vi "Programa_robot_final_7.vi"(8 "error in (no error)":errorcluster) -> (0 "error out":errorcluster={"status"=FALSE, "code"=1073676294, "source"="VISA Read in Programa_robot_final_7.vi"} {"code" format="%f"})   [LabVIEW 2019]
uses:
  <vilib>/Instr/_visa.llb/VISA Configure Serial Port (Instr).vi
  Global_STOP.vi
  <vilib>/regexp/Match Regular Expression.xnode
panel:
  out "FIN BANDEJA ENTRADA":bool
  out "FIN BANDEJA OK":bool
  out "FIN BANDEJA NOK":bool
  out "NUMERO ASICS TESTEADOS":i32=8
  in  "stop socket 3":bool
  in  "Ruta hacia el fichero que contiene la imagen de la       superficie del ASIC  fotografiada por la camara en el bloque de borrado de la imagen previa capturada":path=path "C:/Trabajo_Robot/Test Asic Javi_2021/Origen Socket SERVO_PCB_BUENO_v5 (muchos asics)/capturaQR.jpg"
  in  "stop 6":bool
  in  "Abrir socket 2":bool
  in  "Cerrar socket 2":bool
  in  "Interruptor Error 2":bool
  in  "stop 5":bool
  out "Datos_QR 3":string
  out "Existe foto anterior?":bool
  in  "STOP TEST 3":bool
  in  "Interruptor Error":bool
  in  "Cerrar socket":bool
  in  "Abrir socket":bool
  out "Error_QR":bool=TRUE
  out "return count":u32=1
  out "lectura puerto serie":u32
  out "dato escrito puerto serie":string="0"
  out "TEST OK":bool
  in  "STOP TEST 2":bool
  out "Datos_QR 2":string
  in  "Config File":path=path "C:/Trabajo_Robot/Test Asic Javi_2021/Origen Socket SERVO_PCB_BUENO_v5 (muchos asics)/CONFIG/configuracion_robot_CTAV2022A.test"
  in  "SELECCION DE TEST":string(combo)="COMPLETO"
  in  "?":bool
  out "Boolean":bool
  in  "stop socket 2":bool
  out "Bytes at port 3":u32=1
  in  "IN y":string(combo)="00"
  in  "IN x":string(combo)="00"
  in  "NOK y":string(combo)="00"
  in  "NOK x":string(combo)="00"
  in  "OK y":string(combo)="00"
  in  "OK x":string(combo)="00"
  in  "Operator's name":string(combo)="Iñigo Jorge"
  in  "?":bool
  in  "Fichero de registro":path=path "C:/Trabajo_Robot/QC_LSTSUR/LOG/registro.txt"
  in  "Path Out Report":path=path "C:/Trabajo_Robot/QC_LSTSUR"
  in  "stop socket":bool
  out "Bytes at port 1":u32=1
  out "Iteraciones":i32=9
  out "Lectura buffer":string
  in  "Delay (ms)":dbl=1.0 min=1.0 max=9.0 step=1.0
  out "Bytes at port 2":u32
  in  "Interruptor":bool=TRUE
  in  "stop":bool
  # "SI EL TEST SE RALENTIZA, HAY QUE ABORTAR LABVIEW, PRESIONANDO\nEL BOTÓN DE ABORT, Y DESPUÉS SALIRSE COMPLETAMENTE DE LABVIEW, INCLUYENDO\nCERRAR LA VENTANA GENÉRICA DE LABVIEW QUE NOS SALE DESPUÉS DE QUE SE CIERRE\n\"PROGRAMA_ROBOT_FINAL_7\", PORQUE ES CUANDO LIBERA LA MEMORIA Y DESAPARECEN\nLAS SESIONES VISA y USB QUE NO SE HAN CERRADO AL ABORTAR.\n\nDESPUÉS HAY QUE REINICIAR ARDUINO, DESCONECTANDO Y CONECTANDO EL USB.\n\nCON ÉSTO YA SE PODRÍA VOLVER  A ABRIR EL \"PROGRAMA_ROBOT_FINAL_7\", CON TODO PARTIENDO DE CERO.\n\nEN CUALQUIER OTRA SITUACUÓN QUE PRESIONEMOS EL ABORT DE LABVIEW HAY QUE REALIZAR LA MISMA SECUENCIA."
  # "x: columna en cada bandeja \ny: fila en cada bandeja"
  # "Funcionamiento: en la primera iteración, el efector se desplaza desde el origen hasta la celda\nintroducida, hace una pausa, va a la posición del socket (0,0), hace otra pausa, va a la celda\nde salida y vuelve al origen. En las iteraciones siguientes hará lo mismo pero recorriendo las\nceldas de la bandeja sucesivamente. Que el desplazamiento se produzca hacia una celda de\nla bandeja OK o de la bandeja NOK depende de la salidad del programa de test de Asics."
types:
  T1 = enum16{"open", "replace", "create", "open or create", "replace or create", "replace or create with confirmation"}
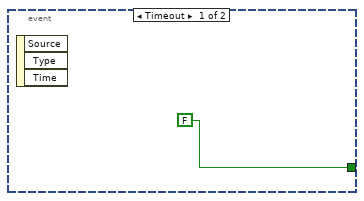
[diagram p2: hidden frame]
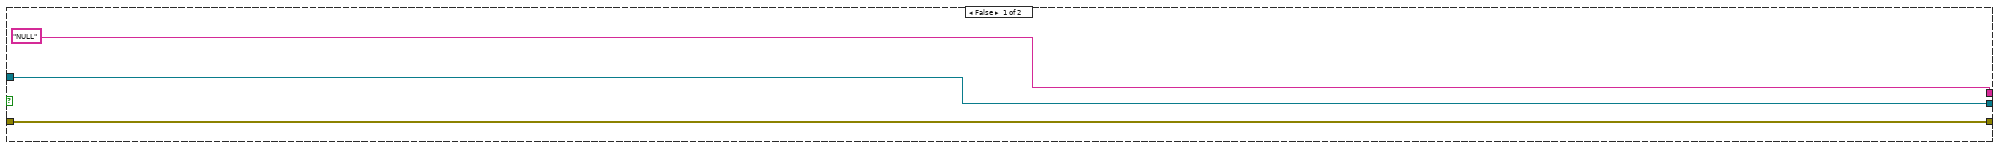
[diagram p5: hidden frame]
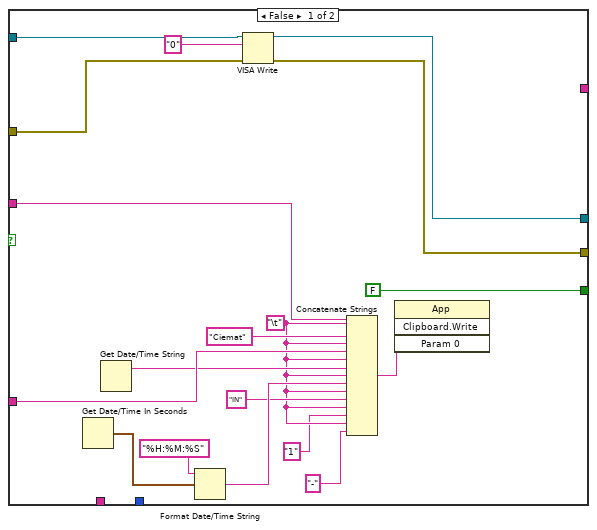
[diagram p9: hidden frame]
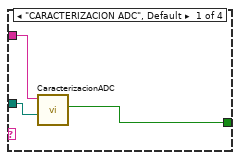
[diagram p10: hidden frame]
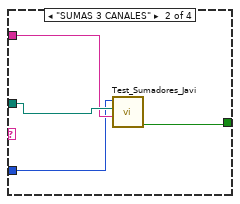
[diagram p11: hidden frame]
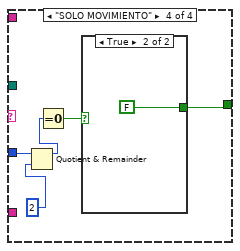
[diagram p12: hidden frame]
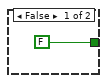
[diagram p13: hidden frame]
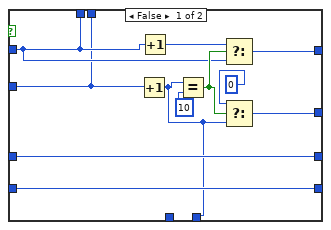
[diagram p15: hidden frame]
diagram:
  # "COORDENADA INICIAL DE \nLA BANDEJA DE ENTRADA"
  n1 = control-ref of="stop socket"() -> (w4:refnum<vi>)
  n2 = control-ref of="Cerrar socket"() -> (w12:refnum<vi>)
  n3 = control-ref of="STOP TEST 2"() -> (w15:refnum<vi>)
  n4 = control-ref of="Abrir socket"() -> (w10:refnum<vi>)
  n5 = control-ref of="stop"() -> (w11:refnum<vi>)
  n6 = control-ref of="Interruptor Error"() -> (w13:refnum<vi>)
  n7 = property class="Bool (strict)"(reference=w15, "Visible"=FALSE) -> ()  [unwired: 1 in, 2 out]
  n8 = property class="Bool (strict)"(reference=w10, "Visible"=FALSE) -> ()  [unwired: 1 in, 2 out]
  n9 = property class="Bool (strict)"(reference=w13, "Visible"=FALSE) -> ()  [unwired: 1 in, 2 out]
  n10 = property class="Bool (strict)"(reference=w12, "Visible"=FALSE) -> ()  [unwired: 1 in, 2 out]
  n11 = property on="Boolean" class="Bool (strict)"("Visible"=FALSE) -> ()  [unwired: 2 in, 2 out]
  n12 = property class="Bool"(reference=w4, "Visible"=FALSE) -> ()  [unwired: 1 in, 2 out]
  n13 = property class="Bool"(reference=w11, "Visible"=FALSE) -> ()  [unwired: 1 in, 2 out]
  n14 = flat-sequence {
    tunnel: [w60] -> w21
    tunnel: ["Fichero de registro"] -> w20
    tunnel: ["SELECCION DE TEST"] -> w19
    tunnel: ["NOK y"] -> w34
    tunnel: ["NOK x"] -> w33
    tunnel: ["OK y"] -> w32
    tunnel: ["OK x"] -> w31
    tunnel: ["IN y"] -> w30
    tunnel: ["IN x"] -> w29
    tunnel: [w63] -> w28
    tunnel: [w64] -> w27
    tunnel: ["IN y"] -> w26
    tunnel: ["IN x"] -> w25
    tunnel: w20 -> [w62]
    frame #0 {
      # "POLLING PARA DETECTAR LA PULSACION\nDEL BOTON DE START"
      n15 = while {
        stop <- "?" stop-if-true
        n16 = property class="Bool"("Visible"=TRUE) -> ()  [unwired: 2 in, 2 out]
        n17 = Not(x="?") -> (.not. x?=w55:bool)
        "Boolean" <- w55
        n18 = property on="Boolean" class="Bool (strict)"("Blinking"=w55) -> ()  [unwired: 2 in, 2 out]
      }
      n19 = property on="FIN BANDEJA ENTRADA" class="Bool (strict)"("Value"=FALSE ("FIN BANDEJA ENTRADA")) -> ()  [unwired: 2 in, 2 out]
      n20 = property on="FIN BANDEJA OK" class="Bool (strict)"("Value"=FALSE ("FIN BANDEJA OK")) -> ()  [unwired: 2 in, 2 out]
      n21 = property on="FIN BANDEJA NOK" class="Bool (strict)"("Value"=FALSE ("FIN BANDEJA NOK")) -> ()  [unwired: 2 in, 2 out]
      n22 = global write "Global_STOP.vi" "stop"(FALSE ("stop")) -> ()
    }
    frame #1 {
      # "BOTON START DESAPARECE"
      n23 = property class="Bool"("Visible"=FALSE) -> ()  [unwired: 2 in, 2 out]
      n24 = Not(x="?") -> (.not. x?=w60:bool)
    }
    frame #2 {
      # "abre el fichero de log donde se registra los asics testeados , resultado del test\noperador , fila y columna de la bandeja donde ha cogido asic , fecha..."
      n25 = Open/Create/Replace File(file path (use dialog)=w62, operation (0:open)=T1."open or create", access (0:read/write)=enum16{"read/write", "read-only", "write-only"}."write-only") -> (refnum out=w75:refnum<file>, error out=w77:errorcluster)  [unwired: 3 in, 1 out]
      n26 = Set File Position(refnum=w75, from (0:start)=enum16{"start", "end", "current"}."end", error in=w77) -> (refnum out=w76:refnum<file>, error out=w78:errorcluster)  [unwired: 1 in]
      n27 = Write to Text File(file (use dialog)=w76, text="\r\n", error in=w78) -> (refnum out=w64:refnum<file>, error out=w63:errorcluster)  [unwired: 1 in, 1 out]
    }
  }
  n28 = Decimal String To Number(string=w26) -> (number=w3:i32)  [unwired: 2 in, 1 out]
  n29 = Decimal String To Number(string=w25) -> (number=w2:i32)  [unwired: 2 in, 1 out]
  n30 = Multiply(x=10, y=w3) -> (x*y=w23:i32)
  n31 = Decimal String To Number(string=w32) -> (number=w36:i32)  [unwired: 2 in, 1 out]
  n32 = Decimal String To Number(string=w31) -> (number=w35:i32)  [unwired: 2 in, 1 out]
  n33 = Decimal String To Number(string=w34) -> (number=w38:i32)  [unwired: 2 in, 1 out]
  n34 = Decimal String To Number(string=w33) -> (number=w37:i32)  [unwired: 2 in, 1 out]
  n35 = call-poly "VISA Configure Serial Port"("VISA resource name"=refnum<visa-resource-name> "COM4", "baud rate (9600)"=u32 9600, "data bits (8)"=u16 8, "error in (no error)"="error in (no error)") -> ("VISA resource name out"=w42:refnum<visa-resource-name>, "error out"=w45:errorcluster)  [unwired: 10 in]
  n36 = Add(x=w23, y=w2) -> (x+y=w22:i32)
  n37 = while {
    shift-right: [w121] -> w43
    shift-left: w45 -> [w156]
    tunnel: w42 -> [w154]
    tunnel: [w123] -> w44
    tunnel: w27 -> [w147]
    tunnel: [w146] -> w41
    tunnel: w28 -> [w145]
    tunnel: [w144] -> w40
    tunnel: w29 -> [w142]
    tunnel: w30 -> [w141]
    tunnel: w31 -> [w140]
    tunnel: w32 -> [w139]
    tunnel: w33 -> [w138]
    tunnel: w34 -> [w137]
    shift-right: [w105] -> _
    shift-left: w38 -> [w136]
    shift-right: [w102] -> _
    shift-left: w37 -> [w135]
    shift-right: [w104] -> _
    shift-left: w36 -> [w134]
    shift-right: [w101] -> _
    shift-left: w35 -> [w133]
    tunnel: w22 -> [w111]
    tunnel: w21 -> [w125]
    tunnel: w19 -> [w124]
    tunnel: [w112] -> w17
    shift-right: [w79] -> _
    shift-left: w3 -> [w89]
    shift-right: [w80] -> _
    shift-left: w2 -> [w88]
    i -> [w109]
    stop <- w110 stop-if-true
    w100 = 10
    w103 = 26 ("y")
    # "Cuando Arduino deja un ASIC en la bandeja de  entrada ó en las de OK/NOK\ny vuelve a la posicion de socket, envia un \"2\" por el puerto serie\na labview y éste lo lee para que se salga del bucle, y prosiga la secuencia que le queda\nal programa, para después coger otro asic. Javier Morales"
    n38 = flat-sequence {
      tunnel: w156 -> [w211]
      tunnel: w154 -> [w200]
      tunnel: [w202] -> w153
      tunnel: [w201] -> w152
      tunnel: w142 -> [w181]
      tunnel: w141 -> [w180]
      tunnel: w140 -> [w179]
      tunnel: w139 -> [w178]
      tunnel: w138 -> [w177]
      tunnel: w137 -> [w176]
      tunnel: w153 -> [w948]
      tunnel: w152 -> [w947]
      tunnel: [w946] -> w132
      tunnel: [w945] -> w130
      tunnel: [w944] -> _
      tunnel: w132 -> [w965]
      tunnel: [w963] -> w131
      tunnel: w130 -> [w964]
      tunnel: [w962] -> w129
      tunnel: w131 -> [w987]
      tunnel: w129 -> [w986]
      tunnel: w109 -> [w988]
      tunnel: [w984] -> w128
      tunnel: [w983] -> w127
      tunnel: [w982] -> w126
      tunnel: [w979] -> w107
      tunnel: w109 -> [w1106]
      tunnel: [w1108] -> w150
      tunnel: [w1107] -> w149
      tunnel: [w1104] -> w143
      tunnel: w128 -> [w1103]
      tunnel: w127 -> [w1102]
      tunnel: w126 -> [w1101]
      tunnel: w125 -> [w1096]
      tunnel: w124 -> [w1099]
      tunnel: w109 -> [w1098]
      tunnel: [w1092] -> w108
      tunnel: w107 -> [w1092]
      tunnel: [w1091] -> w106
      tunnel: [w1190] -> w148
      tunnel: [w1192] -> w151
      tunnel: w150 -> [w1191]
      tunnel: w149 -> [w1189]
      tunnel: w147 -> [w1196]
      tunnel: [w1195] -> w146
      tunnel: w145 -> [w1194]
      tunnel: [w1193] -> w144
      tunnel: w109 -> [w1186]
      tunnel: w143 -> [w1185]
      tunnel: w136 -> [w1181]
      tunnel: w135 -> [w1184]
      tunnel: w134 -> [w1183]
      tunnel: w133 -> [w1182]
      tunnel: [w1180] -> w105
      tunnel: [w1179] -> w102
      tunnel: [w1178] -> w104
      tunnel: [w1177] -> w101
      tunnel: w111 -> [w1176]
      tunnel: w109 -> [w1175]
      tunnel: [w1174] -> _
      tunnel: w108 -> [w1173]
      tunnel: w106 -> [w1172]
      tunnel: [w1171] -> w93
      tunnel: [w1170] -> w92
      tunnel: w89 -> [w1164]
      tunnel: w88 -> [w1169]
      tunnel: [w1166] -> w80
      tunnel: [w1162] -> w79
      tunnel: [w1161] -> w86
      frame #0 {
        n39 = for {
          N: 2 -> [_]
          shift-right: [w823] -> _
          shift-left: w181 -> [w828]
          shift-right: [w826] -> w197
          shift-left: w200 -> [w827]
          shift-right: [w824] -> w196
          shift-left: w211 -> [w825]
          n40 = xnode "Match Regular Expression"("input string"=w828, "regular expression"="-?\\d") -> ("whole match"=w822:string, "after match"=w823:string)  [unwired: 4 in, 3 out]
          n41 = VISA Write(VISA resource name=w827, write buffer=w822, error in (no error)=w825) -> (VISA resource name out=w826:refnum<visa-resource-name>, error out=w824:errorcluster)  [unwired: 1 out]
        }
        n42 = for {
          N: 2 -> [_]
          shift-right: [w701] -> _
          shift-left: w180 -> [w706]
          shift-right: [w704] -> w191
          shift-left: w197 -> [w705]
          shift-right: [w702] -> w190
          shift-left: w196 -> [w703]
          n43 = xnode "Match Regular Expression"("input string"=w706, "regular expression"="-?\\d") -> ("whole match"=w700:string, "after match"=w701:string)  [unwired: 4 in, 3 out]
          n44 = VISA Write(VISA resource name=w705, write buffer=w700, error in (no error)=w703) -> (VISA resource name out=w704:refnum<visa-resource-name>, error out=w702:errorcluster)  [unwired: 1 out]
        }
        n45 = for {
          N: 2 -> [_]
          shift-right: [w579] -> _
          shift-left: w179 -> [w584]
          shift-right: [w582] -> w193
          shift-left: w191 -> [w583]
          shift-right: [w580] -> w192
          shift-left: w190 -> [w581]
          n46 = xnode "Match Regular Expression"("input string"=w584, "regular expression"="-?\\d") -> ("whole match"=w578:string, "after match"=w579:string)  [unwired: 4 in, 3 out]
          n47 = VISA Write(VISA resource name=w583, write buffer=w578, error in (no error)=w581) -> (VISA resource name out=w582:refnum<visa-resource-name>, error out=w580:errorcluster)  [unwired: 1 out]
        }
        n48 = for {
          N: 2 -> [_]
          shift-right: [w457] -> _
          shift-left: w178 -> [w462]
          shift-right: [w460] -> w185
          shift-left: w193 -> [w461]
          shift-right: [w458] -> w184
          shift-left: w192 -> [w459]
          n49 = xnode "Match Regular Expression"("input string"=w462, "regular expression"="-?\\d") -> ("whole match"=w456:string, "after match"=w457:string)  [unwired: 4 in, 3 out]
          n50 = VISA Write(VISA resource name=w461, write buffer=w456, error in (no error)=w459) -> (VISA resource name out=w460:refnum<visa-resource-name>, error out=w458:errorcluster)  [unwired: 1 out]
        }
        n51 = for {
          N: 2 -> [_]
          shift-right: [w335] -> _
          shift-left: w177 -> [w340]
          shift-right: [w338] -> w187
          shift-left: w185 -> [w339]
          shift-right: [w336] -> w186
          shift-left: w184 -> [w337]
          n52 = xnode "Match Regular Expression"("input string"=w340, "regular expression"="-?\\d") -> ("whole match"=w334:string, "after match"=w335:string)  [unwired: 4 in, 3 out]
          n53 = VISA Write(VISA resource name=w339, write buffer=w334, error in (no error)=w337) -> (VISA resource name out=w338:refnum<visa-resource-name>, error out=w336:errorcluster)  [unwired: 1 out]
        }
        n54 = for {
          N: 2 -> [_]
          shift-right: [w213] -> _
          shift-left: w176 -> [w218]
          shift-right: [w216] -> w183
          shift-left: w187 -> [w217]
          shift-right: [w214] -> w182
          shift-left: w186 -> [w215]
          n55 = xnode "Match Regular Expression"("input string"=w218, "regular expression"="-?\\d") -> ("whole match"=w212:string, "after match"=w213:string)  [unwired: 4 in, 3 out]
          n56 = VISA Write(VISA resource name=w217, write buffer=w212, error in (no error)=w215) -> (VISA resource name out=w216:refnum<visa-resource-name>, error out=w214:errorcluster)  [unwired: 1 out]
        }
        n57 = Number To Decimal String(number="Delay (ms)") -> (decimal integer string=w205:string)  [unwired: 1 in]
        n58 = VISA Write(VISA resource name=w183, write buffer=w205, error in (no error)=w182) -> (VISA resource name out=w207:refnum<visa-resource-name>, error out=w206:errorcluster)  [unwired: 1 out]
        n59 = Select(t="1" ("write buffer"), s="Interruptor", f="0" ("write buffer")) -> (s? t:f=w203:string)
        n60 = VISA Write(VISA resource name=w207, write buffer=w203, error in (no error)=w206) -> (VISA resource name out=w202:refnum<visa-resource-name>, error out=w201:errorcluster)  [unwired: 1 out]
      }
      frame #1 {
        n61 = while {
          shift-right: [w955] -> w945
          shift-left: w947 -> [w960]
          tunnel: ["stop socket"] -> _
          shift-right: [w956] -> w946
          shift-left: w948 -> [w961]
          tunnel: ["stop socket"] -> w944
          stop <- w950 stop-if-true
          n62 = property class="Instr"(reference=w961, error in=w960) -> (reference out=w959:refnum<visa-resource-name>, error out=w958:errorcluster, "Bytes at Port"=w957:u32)
          "Bytes at port 1" <- w957
          n63 = VISA Read(VISA resource name=w959, byte count=w957, error in (no error)=w958) -> (VISA resource name out=w956:refnum<visa-resource-name>, read buffer=w954:string, error out=w955:errorcluster)  [unwired: 1 out]
          n64 = Equal?(x="2", y=w954) -> (x = y?=w952:bool)
          n65 = global read "Global_STOP.vi" "stop"() -> (w949:bool)
          n66 = Compound Arithmetic op=OR(w952, "stop socket", w949) -> (w950:bool)
        }
      }
      frame #2 {
        n67 = while {
          shift-right: [w972] -> w962
          shift-left: w964 -> [w977]
          tunnel: ["stop socket 2"] -> _
          shift-right: [w973] -> w963
          shift-left: w965 -> [w978]
          tunnel: ["stop socket 2"] -> _
          stop <- w967 stop-if-true
          n68 = property class="Instr"(reference=w978, error in=w977) -> (reference out=w976:refnum<visa-resource-name>, error out=w975:errorcluster, "Bytes at Port"=w974:u32)
          "Bytes at port 3" <- w974
          n69 = VISA Read(VISA resource name=w976, byte count=w974, error in (no error)=w975) -> (VISA resource name out=w973:refnum<visa-resource-name>, read buffer=w971:string, error out=w972:errorcluster)  [unwired: 1 out]
          n70 = Equal?(x="3", y=w971) -> (x = y?=w969:bool)
          n71 = global read "Global_STOP.vi" "stop"() -> (w966:bool)
          n72 = Compound Arithmetic op=OR(w969, "stop socket 2", w966) -> (w967:bool)
        }
      }
      frame #3 {
        # "Este bloque realiza la captura y lectura del QR"
        n73 = Greater?(x=w988, y=-1) -> (0:w985:bool)
        n74 = case shown="True" w985 {
          tunnel: [w992 w995] -> w982
          tunnel: w987 -> [w992 w997]
          tunnel: [w991 w996] -> w984
          tunnel: w986 -> [w991 w998]
          tunnel: ["NULL" ("Datos_QR") w994] -> w983
          frame False {
          }
          frame True {
            n75 = property on="Error_QR" class="Bool (strict)"("Value"=FALSE ("Error_QR")) -> ()  [unwired: 2 in, 2 out]
            n76 = while {
              tunnel: [w1005] -> w994
              tunnel: w997 -> [w1015]
              tunnel: [w1011] -> w995
              tunnel: [w1010] -> w996
              tunnel: w998 -> [w1006]
              stop <- w1003 stop-if-true
              n77 = flat-sequence {
                tunnel: [w1019] -> w1007
                tunnel: w1006 -> [w1017]
                tunnel: [w1031] -> w1005
                tunnel: [w1030] -> w1000
                tunnel: w1007 -> [w1029]
                tunnel: [w1029] -> w1001
                frame #0 {
                  # "Éste bloque borra el fichero de imagen\ndel Asic anterior."
                  n78 = call <vilib>:"Check if File or Folder Exists.vi"("error in (no error)"=w1017, "path"="Ruta hacia el fichero que contiene la imagen de la       superficie del ASIC  fotografiada por la camara en el bloque de borrado de la imagen previa capturada") -> ("error out"=w1018:errorcluster, "file or folder exists?"=w1021:bool, "dup path"=w1020:path)  [unwired: 7 in]
                  "Existe foto anterior?" <- w1021
                  n79 = case shown="True" w1021 {
                    tunnel: w1020 -> [w1023 w1027]
                    tunnel: [w1023 w1026] -> _
                    tunnel: [w1022 w1025] -> w1019
                    tunnel: w1018 -> [w1022 w1024]
                    frame False {
                    }
                    frame True {
                      n80 = Delete(path (use dialog)=w1027, error in=w1024) -> (deleted path=w1026:path, error out=w1025:errorcluster)  [unwired: 3 in, 1 out]
                    }
                  }
                }
                frame #1 {
                  # "Éste bloque realiza la captura de imagen\ndel QR del Asic para leer el código."
                  n81 = for {
                    N: 5 -> [_]
                    tunnel: [w1036] -> w1031
                    tunnel: [w1034] -> w1030
                    stop <- w1032 stop-if-true
                    n82 = call "CapturaImagenyQR_subVI_pruebas.vi"() -> ("Datos_QR"=w1036:string)  [unwired: 11 in]
                    "Datos_QR 3" <- w1036
                    n83 = Equal?(x=w1036, y="" ("Datos_QR")) -> (x = y?=w1035:bool)
                    n84 = global read "Global_STOP.vi" "stop"() -> (w1033:bool)
                    n85 = Not(x=w1035) -> (.not. x?=w1034:bool)
                    n86 = Compound Arithmetic op=OR(w1034, w1033) -> (w1032:bool)
                  }
                }
              }
              n87 = Not(x=w1000) -> (.not. x?=w1002:bool)
              "Error_QR" <- w1002
              n88 = Select(t="1" ("write buffer"), s=w1000, f="0" ("write buffer")) -> (s? t:f=w1012:string)
              n89 = VISA Write(VISA resource name=w1015, write buffer=w1012, error in (no error)=w1001) -> (VISA resource name out=w1009:refnum<visa-resource-name>, error out=w1008:errorcluster)  [unwired: 1 out]
              n90 = global read "Global_STOP.vi" "stop"() -> (w1004:bool)
              n91 = case shown="False" w1000 {
                tunnel: w1009 -> [w1049 w1090]
                tunnel: w1008 -> [w1048 w1089]
                tunnel: [w1047 w1090] -> w1011
                tunnel: [w1046 w1089] -> w1010
                frame False {
                  n92 = flat-sequence {
                    tunnel: w1049 -> [w1053]
                    tunnel: [w1052] -> w1045
                    tunnel: [w1051] -> w1043
                    tunnel: w1048 -> [w1050]
                    tunnel: w1045 -> [w1066]
                    tunnel: [w1066] -> w1044
                    tunnel: w1043 -> [w1065]
                    tunnel: [w1065] -> w1042
                    tunnel: w1044 -> [w1070]
                    tunnel: w1042 -> [w1069]
                    tunnel: [w1068] -> w1041
                    tunnel: [w1067] -> w1039
                    tunnel: w1041 -> [w1083]
                    tunnel: [w1083] -> w1040
                    tunnel: w1039 -> [w1082]
                    tunnel: [w1082] -> w1038
                    tunnel: [w1084] -> w1046
                    tunnel: [w1085] -> w1047
                    tunnel: w1040 -> [w1085]
                    tunnel: w1038 -> [w1084]
                    frame #0 {
                      n93 = while {
                        tunnel: w1053 -> [w1063]
                        tunnel: [w1059] -> w1052
                        tunnel: [w1058] -> w1051
                        tunnel: w1050 -> [w1057]
                        stop <- w1054 stop-if-true
                        n94 = global read "Global_STOP.vi" "stop"() -> (w1056:bool)
                        n95 = Select(t="2" ("write buffer"), s="Abrir socket", f="0" ("write buffer")) -> (s? t:f=w1060:string)
                        n96 = Or(x=w1056, y="Abrir socket") -> (x .or. y?=w1054:bool)
                        n97 = VISA Write(VISA resource name=w1063, write buffer=w1060, error in (no error)=w1057) -> (VISA resource name out=w1059:refnum<visa-resource-name>, error out=w1058:errorcluster)  [unwired: 1 out]
                      }
                    }
                    frame #1 {
                      n98 = Wait (ms)(milliseconds to wait=u32 1000) -> ()  [unwired: 1 out]
                    }
                    frame #2 {
                      n99 = while {
                        tunnel: w1070 -> [w1077]
                        tunnel: w1069 -> [w1076]
                        tunnel: [w1075] -> w1068
                        tunnel: [w1074] -> w1067
                        stop <- w1073 stop-if-true
                        n100 = global read "Global_STOP.vi" "stop"() -> (w1072:bool)
                        n101 = Select(t="3" ("write buffer"), s="Cerrar socket", f="0" ("write buffer")) -> (s? t:f=w1078:string)
                        n102 = Or(x=w1072, y="Cerrar socket") -> (x .or. y?=w1073:bool)
                        n103 = VISA Write(VISA resource name=w1077, write buffer=w1078, error in (no error)=w1076) -> (VISA resource name out=w1075:refnum<visa-resource-name>, error out=w1074:errorcluster)  [unwired: 1 out]
                      }
                    }
                    frame #3 {
                      n104 = Wait (ms)(milliseconds to wait=u32 1000) -> ()  [unwired: 1 out]
                    }
                    frame #4 {
                      n105 = while {
                        stop <- w1086 stop-if-true
                        n106 = global read "Global_STOP.vi" "stop"() -> (w1088:bool)
                        n107 = Or(x="Interruptor Error", y=w1088) -> (x .or. y?=w1086:bool)
                      }
                    }
                  }
                }
                frame True {
                }
              }
              n108 = Or(x=w1000, y=w1004) -> (x .or. y?=w1003:bool)
              n109 = case shown="True" w1002 {
                frame False {
                }
                frame True {
                  n110 = call "Send Email"() -> ()  [unwired: 11 in, 1 out]
                }
              }
            }
            n111 = Wait (ms)(milliseconds to wait=u32 10000) -> ()  [unwired: 1 out]
          }
        }
        n112 = control-ref of="STOP TEST 2"() -> (w981:refnum<vi>)
        n113 = property class="Bool (strict)"(reference=w981, "Visible"=TRUE) -> ()  [unwired: 1 in, 2 out]
        n114 = Get Date/Time In Seconds() -> (seconds since 1Jan1904=w979:timestamp)
      }
      frame #4 {
        n115 = global read "Global_STOP.vi" "stop"() -> (w1095:bool)
        n116 = Greater?(x=w1106, y=-1) -> (0:w1097:bool)
        n117 = Not(x=w1095) -> (.not. x?=w1094:bool)
        n118 = Compound Arithmetic op=AND(w1097, w1096, w1094) -> (w1093:bool)
        n119 = case shown="True" w1093 {
          tunnel: w1101 -> [w1124 w1133]
          tunnel: w1103 -> [w1123 w1132]
          tunnel: [w1122 w1131] -> w1108
          tunnel: [w1121 w1130] -> w1107
          tunnel: w1102 -> [w1117 w1127]
          tunnel: [FALSE ("Boolean") w1137] -> w1104
          tunnel: "Operator's name" -> [w1115 w1136]
          tunnel: w1099 -> [_ w1128]
          tunnel: w1098 -> [_ w1135]
          tunnel: [_ w1127] -> w1091
          frame False {
            w1111 = "\t"
            n120 = Get Date/Time In Seconds() -> (seconds since 1Jan1904=w1119:timestamp)
            n121 = Get Date/Time String() -> (date string=w1114:string)  [unwired: 3 in, 1 out]
            n122 = Format Date/Time String(time format string (%c)="%H:%M:%S", seconds (now)=w1119) -> (date/time string=w1113:string)  [unwired: 1 in]
            n123 = VISA Write(VISA resource name=w1124, write buffer="0", error in (no error)=w1123) -> (VISA resource name out=w1122:refnum<visa-resource-name>, error out=w1121:errorcluster)  [unwired: 1 out]
            n124 = Concatenate Strings(w1117, w1111, "Ciemat", w1111, w1115, w1111, w1114, w1111, w1113, w1111, "IN", w1111, "1", w1111, "-") -> (w1120:string)
            n125 = invoke class="App" method="Clipboard.Write"("Param 0"=w1120) -> ()  [unwired: 3 in, 4 out]
          }
          frame True {
            # "Test de Asics"
            n126 = case shown="\"COMPLETO\"" w1128 {
              tunnel: w1127 -> [w1143 w1145 w1153 _]
              tunnel: "Path Out Report" -> [w1142 w1147 w1151 _]
              tunnel: [w1141 w1146 w1149 w1154] -> w1137
              tunnel: w1136 -> [_ _ w1152 _]
              tunnel: w1135 -> [_ w1144 w1148 w1158]
              frame "CARACTERIZACION ADC", Default {
                n127 = call "CaracterizacionADC.vi"("QR code"=w1143, "Path Out Report"=w1142) -> ("OK/NOK"=w1141:bool)  [unwired: 7 in]
              }
              frame "SUMAS 3 CANALES" {
                n128 = call "Test_Sumadores_Javi.vi"("QR"=w1145, "Path"=w1147, "NUMERO DE PASADA DE TEST"=w1144) -> ("Boolean"=w1146:bool)  [unwired: 8 in]
              }
              frame "COMPLETO" {
                n129 = call "Test Asic V1.0_2019_2.vi"("Config File"="Config File", "Path Out Report"=w1151, "Operator's Name"=w1152, "ASIC'S Number"=w1153) -> ("OK, Fault 2"=w1149:bool)  [unwired: 1 in]
                "NUMERO ASICS TESTEADOS" <- w1148
              }
              frame "SOLO MOVIMIENTO" {
                n130 = Quotient & Remainder(x=w1158, y=2) -> (x-y*floor(x/y)=w1155:i32)  [unwired: 1 out]
                n131 = Equal To 0?(x=w1155) -> (x = 0?=w1156:bool)
                n132 = case shown="True" w1156 {
                  tunnel: [FALSE FALSE] -> w1154
                  frame False {
                  }
                  frame True {
                  }
                }
              }
            }
            "TEST OK" <- w1137
            n133 = Select(t="1" ("write buffer"), s=w1137, f="0" ("write buffer")) -> (s? t:f=w1134:string)
            "dato escrito puerto serie" <- w1134
            n134 = VISA Write(VISA resource name=w1133, write buffer=w1134, error in (no error)=w1132) -> (VISA resource name out=w1131:refnum<visa-resource-name>, return count=→"return count":u32, error out=w1130:errorcluster)
          }
        }
      }
      frame #5 {
        n135 = Greater?(x=w1186, y=-1) -> (0:w1187:bool)
        n136 = case shown="True" w1187 {
          tunnel: w1196 -> [w1202 w1207]
          tunnel: [w1202 w1208] -> w1195
          tunnel: w1194 -> [w1201 w1210]
          tunnel: [w1201 w1209] -> w1193
          tunnel: [w1204 w1228] -> w1192
          tunnel: w1191 -> [w1204 w1228]
          tunnel: [w1203 w1227] -> w1190
          tunnel: w1189 -> [w1203 w1227]
          tunnel: w1185 -> [_ w1213]
          tunnel: w1181 -> [w1200 w1226]
          tunnel: w1184 -> [w1199 w1225]
          tunnel: w1183 -> [w1198 w1224]
          tunnel: w1182 -> [w1197 w1223]
          tunnel: [w1200 w1222] -> w1180
          tunnel: [w1199 w1221] -> w1179
          tunnel: [w1198 w1220] -> w1178
          tunnel: [w1197 w1219] -> w1177
          tunnel: [_ w1214] -> _
          tunnel: w1173 -> [_ w1214]
          tunnel: w1172 -> [_ w1211]
          tunnel: [_ w1206] -> w1171
          tunnel: [_ w1205] -> w1170
          frame False {
          }
          frame True {
            # "Registro de datos en fichero"
            n137 = property on="Operator's name" class="CmbBox"() -> ("Value"=w1212:string)  [unwired: 2 in, 2 out]
            n138 = case shown="True" w1213 {
              tunnel: w1226 -> [w1231 w1244]
              tunnel: w1225 -> [w1230 w1243]
              tunnel: w1224 -> [w1233 w1241]
              tunnel: w1223 -> [w1232 w1242]
              tunnel: [w1235 w1244] -> w1222
              tunnel: [w1234 w1243] -> w1221
              tunnel: [w1233 w1246] -> w1220
              tunnel: [w1232 w1245] -> w1219
              tunnel: [w1231 w1241] -> w1218
              tunnel: [w1230 w1242] -> w1217
              tunnel: [_ w1240] -> w1206
              tunnel: [w1229 _] -> w1205
              frame False {
                n139 = Increment(x=w1230) -> (x+1=w1229:i32)
                n140 = Increment(x=w1231) -> (x+1=w1236:i32)
                n141 = Equal?(x=w1229, y=10) -> (x = y?=w1237:bool)
                n142 = Select(t=w1236, s=w1237, f=w1231) -> (s? t:f=w1235:i32)
                n143 = Select(t=0, s=w1237, f=w1229) -> (s? t:f=w1234:i32)
              }
              frame True {
                n144 = Increment(x=w1242) -> (x+1=w1240:i32)
                n145 = Increment(x=w1241) -> (x+1=w1247:i32)
                n146 = Equal?(x=w1240, y=10) -> (x = y?=w1248:bool)
                n147 = Select(t=w1247, s=w1248, f=w1241) -> (s? t:f=w1246:i32)
                n148 = Select(t=0, s=w1248, f=w1240) -> (s? t:f=w1245:i32)
              }
            }
            n149 = Number To Decimal String(number=w1218) -> (decimal integer string=w1216:string)  [unwired: 1 in]
            n150 = Number To Decimal String(number=w1217) -> (decimal integer string=w1215:string)  [unwired: 1 in]
            n151 = call "Escribir_Fichero_Registro.vi"("refnum FILE"=w1207, "ASIC QR CODE"=w1211, "HORA COMIENZO"=w1214, "Coordenada X"=w1215, "Coordenada Y"=w1216, "OPERADOR"=w1212, "Resultado test"=w1213, "error in (no error)"=w1210) -> ("refnum out"=w1208:refnum<file>, "error out"=w1209:errorcluster)  [unwired: 18 in]
          }
        }
        n152 = Increment(x=w1164) -> (x+1=w1165:i32)
        n153 = Increment(x=w1169) -> (x+1=w1161:i32)
        n154 = Equal?(x=w1161, y=10) -> (x = y?=w1163:bool)
        n155 = Select(t=i16 0, s=w1163, f=w1161) -> (s? t:f=w1166:i32)
        n156 = Select(t=w1165, s=w1163, f=w1164) -> (s? t:f=w1162:i32)
        n157 = Add(x=w1176, y=w1175) -> (x+y=w1174:i32)
      }
    }
    n158 = while {
      shift-right: [w1258] -> w116
      shift-left: w148 -> [w1264]
      tunnel: ["stop"] -> _
      shift-right: [w1259] -> w123
      shift-left: w151 -> [w1265]
      tunnel: [w1254] -> w155
      stop <- w1252 stop-if-true
      # "1"
      n159 = property class="Instr"(reference=w1265, error in=w1264) -> (reference out=w1262:refnum<visa-resource-name>, error out=w1261:errorcluster, "Bytes at Port"=w1260:u32)
      "Bytes at port 2" <- w1260
      n160 = VISA Read(VISA resource name=w1262, byte count=w1260, error in (no error)=w1261) -> (VISA resource name out=w1259:refnum<visa-resource-name>, read buffer=w1254:string, return count=w1257:u32, error out=w1258:errorcluster)
      "lectura puerto serie" <- w1257
      n161 = Greater Or Equal?(x=w1257, y=u32 1) -> (x >= y?=w1255:bool)
      n162 = global read "Global_STOP.vi" "stop"() -> (w1251:bool)
      n163 = Or(x=w1255, y="stop") -> (x .or. y?=w1253:bool)
      n164 = Compound Arithmetic op=OR(w1253, w1251) -> (w1252:bool)
    }
    "Lectura buffer" <- w155
    n165 = Equal?(x=w104, y=w103) -> (x = y?=w97:bool)
    n166 = Equal?(x=w105, y=w103) -> (x = y?=w99:bool)
    n167 = Equal?(x=w92, y=w100) -> (x = y?=w98:bool)
    n168 = Equal?(x=w93, y=w100) -> (x = y?=w96:bool)
    n169 = Equal?(x=w79, y=26) -> (x = y?=w84:bool)
    n170 = Equal?(x=w86, y=10) -> (x = y?=w83:bool)
    n171 = And(x=w99, y=w98) -> (x .and. y?=w95:bool)
    "FIN BANDEJA NOK" <- w95
    n172 = And(x=w84, y=w83) -> (x .and. y?=w82:bool)
    "FIN BANDEJA ENTRADA" <- w82
    n173 = And(x=w97, y=w96) -> (x .and. y?=w94:bool)
    "FIN BANDEJA OK" <- w94
    n174 = Or(x=w95, y=w94) -> (x .or. y?=w90:bool)
    n175 = flat-sequence {
      tunnel: w116 -> [w158]
      tunnel: [w158] -> w115
      tunnel: [w157] -> w113
      frame #0 {
        n176 = global read "Global_STOP.vi" "stop"() -> (w157:bool)
      }
    }
    n177 = case shown="False" w113 {
      selector: w113 -> [_ w168]
      tunnel: [w162 _] -> w120
      tunnel: [w159 w168] -> w117
      tunnel: w115 -> [w160 w167]
      tunnel: [w160 w167] -> w114
      frame False {
        n178 = for {
          N: 3 -> [_]
          tunnel: [w165] -> _
          tunnel: [w163] -> w162
          tunnel: [w163] -> w159
          stop <- w163 stop-if-true
          n179 = call "CapturaImagenyQR_subVI_pruebas.vi"() -> ("Datos_QR"=w165:string)  [unwired: 11 in]
          "Datos_QR 2" <- w165
          n180 = Equal?(x=w165, y="" ("Datos_QR")) -> (x = y?=w164:bool)
          n181 = Not(x=w164) -> (.not. x?=w163:bool)
        }
      }
      frame True {
      }
    }
    n182 = flat-sequence {
      tunnel: [w173] -> w112
      tunnel: w117 -> [w171]
      tunnel: [w170] -> w91
      tunnel: w90 -> [w170]
      tunnel: w82 -> [w169]
      tunnel: [w169] -> w81
      frame #0 {
        n183 = global read "Global_STOP.vi" "stop"() -> (w172:bool)
        n184 = Or(x=w171, y=w172) -> (x .or. y?=w173:bool)
      }
    }
    n185 = Boolean To (0,1)(Boolean=w120) -> (0, 1=w119:i16)
    n186 = call <vilib>:"Error Cluster From Error Code.vi"("error in (no error)"=w114, "error message (\"\")"="El asic no se ha colocado en la\n    bandeja de salida,se ha quedado\nen el socket posiblemente por una\nmala succión de la ventosa.\nPresione STOP\n" ("error message (\"\")"), "error code (0)"=w119) -> ("error out"=w118:errorcluster)  [unwired: 6 in]
    n187 = call <vilib>:"Simple Error Handler.vi"("error in (no error)"=w118) -> ("error out"=w121:errorcluster)  [unwired: 4 in, 4 out]
    n188 = Compound Arithmetic op=OR(w112, w91, w81) -> (w110:bool)
    n189 = case shown="True" w120 {
      selector: w120 -> [w174 w175]
      tunnel: [w174 w175] -> _
      frame False {
      }
      frame True {
        n190 = call "Send Email2"() -> ()  [unwired: 11 in, 1 out]
      }
    }
    "Iteraciones" <- w109
  }
  n191 = flat-sequence {
    frame #0 {
      n192 = local write "STOP TEST 2"(FALSE ("STOP TEST 2")) -> ()
    }
    frame #1 {
      n193 = while {
        stop <- w1267 stop-if-true
        n194 = event shown="[1] \"STOP TEST 2\": Value Change" {
          selector: _ -> [_ _]
          dyn-events: _ -> [_ _]
          timeout: _ -> [_ _]
          tunnel: [FALSE "STOP TEST 2"] -> w1267
          event Timeout {
            n195 = event-data() -> ()  [unwired: 1 in, 3 out]
          }
          event "STOP TEST 2": Value Change {
            n196 = event-data() -> ()  [unwired: 1 in, 6 out]
            n197 = global write "Global_STOP.vi" "stop"("STOP TEST 2") -> ()
            n198 = Wait (ms)(milliseconds to wait=u32 100) -> ()  [unwired: 1 out]
          }
        }
      }
    }
  }
  n199 = Close File(refnum=w41, error in=w40) -> (error out=w39:errorcluster)  [unwired: 1 out]
  n200 = Not(x=w17) -> (.not. x?=w18:bool)
  n201 = call <vilib>:"Simple Error Handler.vi"("error in (no error)"=w39) -> ()  [unwired: 4 in, 5 out]
  n202 = global write "Global_STOP.vi" "stop"(w18) -> ()
  n203 = VISA Close(VISA resource name=w44, error in (no error)=w43) -> (error out=→"error out":errorcluster)
